vi "Processing Test.vi"(8 "Error In":errorcluster, 11 "File Path Control":path=path "C:/Data/Spectra for Fedor/Ok spectra/300.00000K_175_555_2.10000V_0.00000T_May20-2015__09-37-18_001_052015.tdms") -> (0 "Error Out":errorcluster)   [LabVIEW 2016]
uses:
  LabActor/Post-Processors/Line Detector/Line Detector Configuration.ctl
  <vilib>/Analysis/3filter.llb/Filter Passband Type.ctl
  <vilib>/Analysis/3filter.llb/Bessel Filter (CDB).vi
  Utilities/Fit/Smooth Background CDBL.vi
  <vilib>/addons/Wavelet Analysis/application.llb/WA Denoise (DWT Real Array).vi
  <vilib>/addons/Wavelet Analysis/application.llb/WA Detrend (Array).vi
  <vilib>/addons/Wavelet Analysis/application.llb/WA Multiscale Peak Detection (Array).vi
  <vilib>/Analysis/NI_AALPro.lvlib
  <vilib>/Analysis/NI_AAL_SigProc.lvlib
  <vilib>/Analysis/NI_AALBase.lvlib
  <vilib>/addons/_Advanced Signal Processing/NI_AdvSigProcWA.lvlib
panel:
  out "Waveform Graph":dbl[][](graph)
  in  "ASPT?":bool
  out "# found":i32
  out "error":i32
  in  "Low pass distortion":dbl
  out "XY Graph 6":cluster{dbl[], dbl[]}[](graph)
  in  "User configuration":T1={"Peak width"=30.0, "Background removal"=enum."NONE", "Smoothing"=enum."NONE", "Smooth points"=100.0, "Relative threshold"=0.0, "Peak detector"=enum."Normal", "Bgd points"=100.0} {"Bgd points" format="%#_6p"; "Relative threshold" format="%#_6p"; "Peak width" format="%#_6pHz"}
  in  "Signal channel":string="Signal"
  in  "Frequency channel":string="Frequency"
  in  "group name in":string="p"
  in  "HP F":dbl=0.1 format="%#_6p"
  out "LP  F":dbl=0.001 format="%#_6p"
  in  "Fit?":bool
  in  "Complex":bool
  in  "Deviations":dbl=1.0
  out "variance":dbl format="%.2p"
  out "standard deviation":dbl format="%.2p"
  out "Peak F":dbl format="%#_6pHz"
  out "Points around peak":i32=100
  in  "Peak number":i32
  out "XY Graph 5":cluster{"Array":dbl[], "Array":dbl[]}[](graph)
  out "width":i32=100 min=3
  out "XY Graph 4":cluster{"Y":dbl[], dbl[]}(graph)
  out "XY Graph 3":cluster{"Y":dbl[], "Y":dbl[]}[](graph)
  out "Magnitude":cluster{"Y":dbl[], dbl[]}[](graph)
  out "Phase":cluster{"Y":dbl[], "Unwrapped Phase":dbl[]}[](graph)
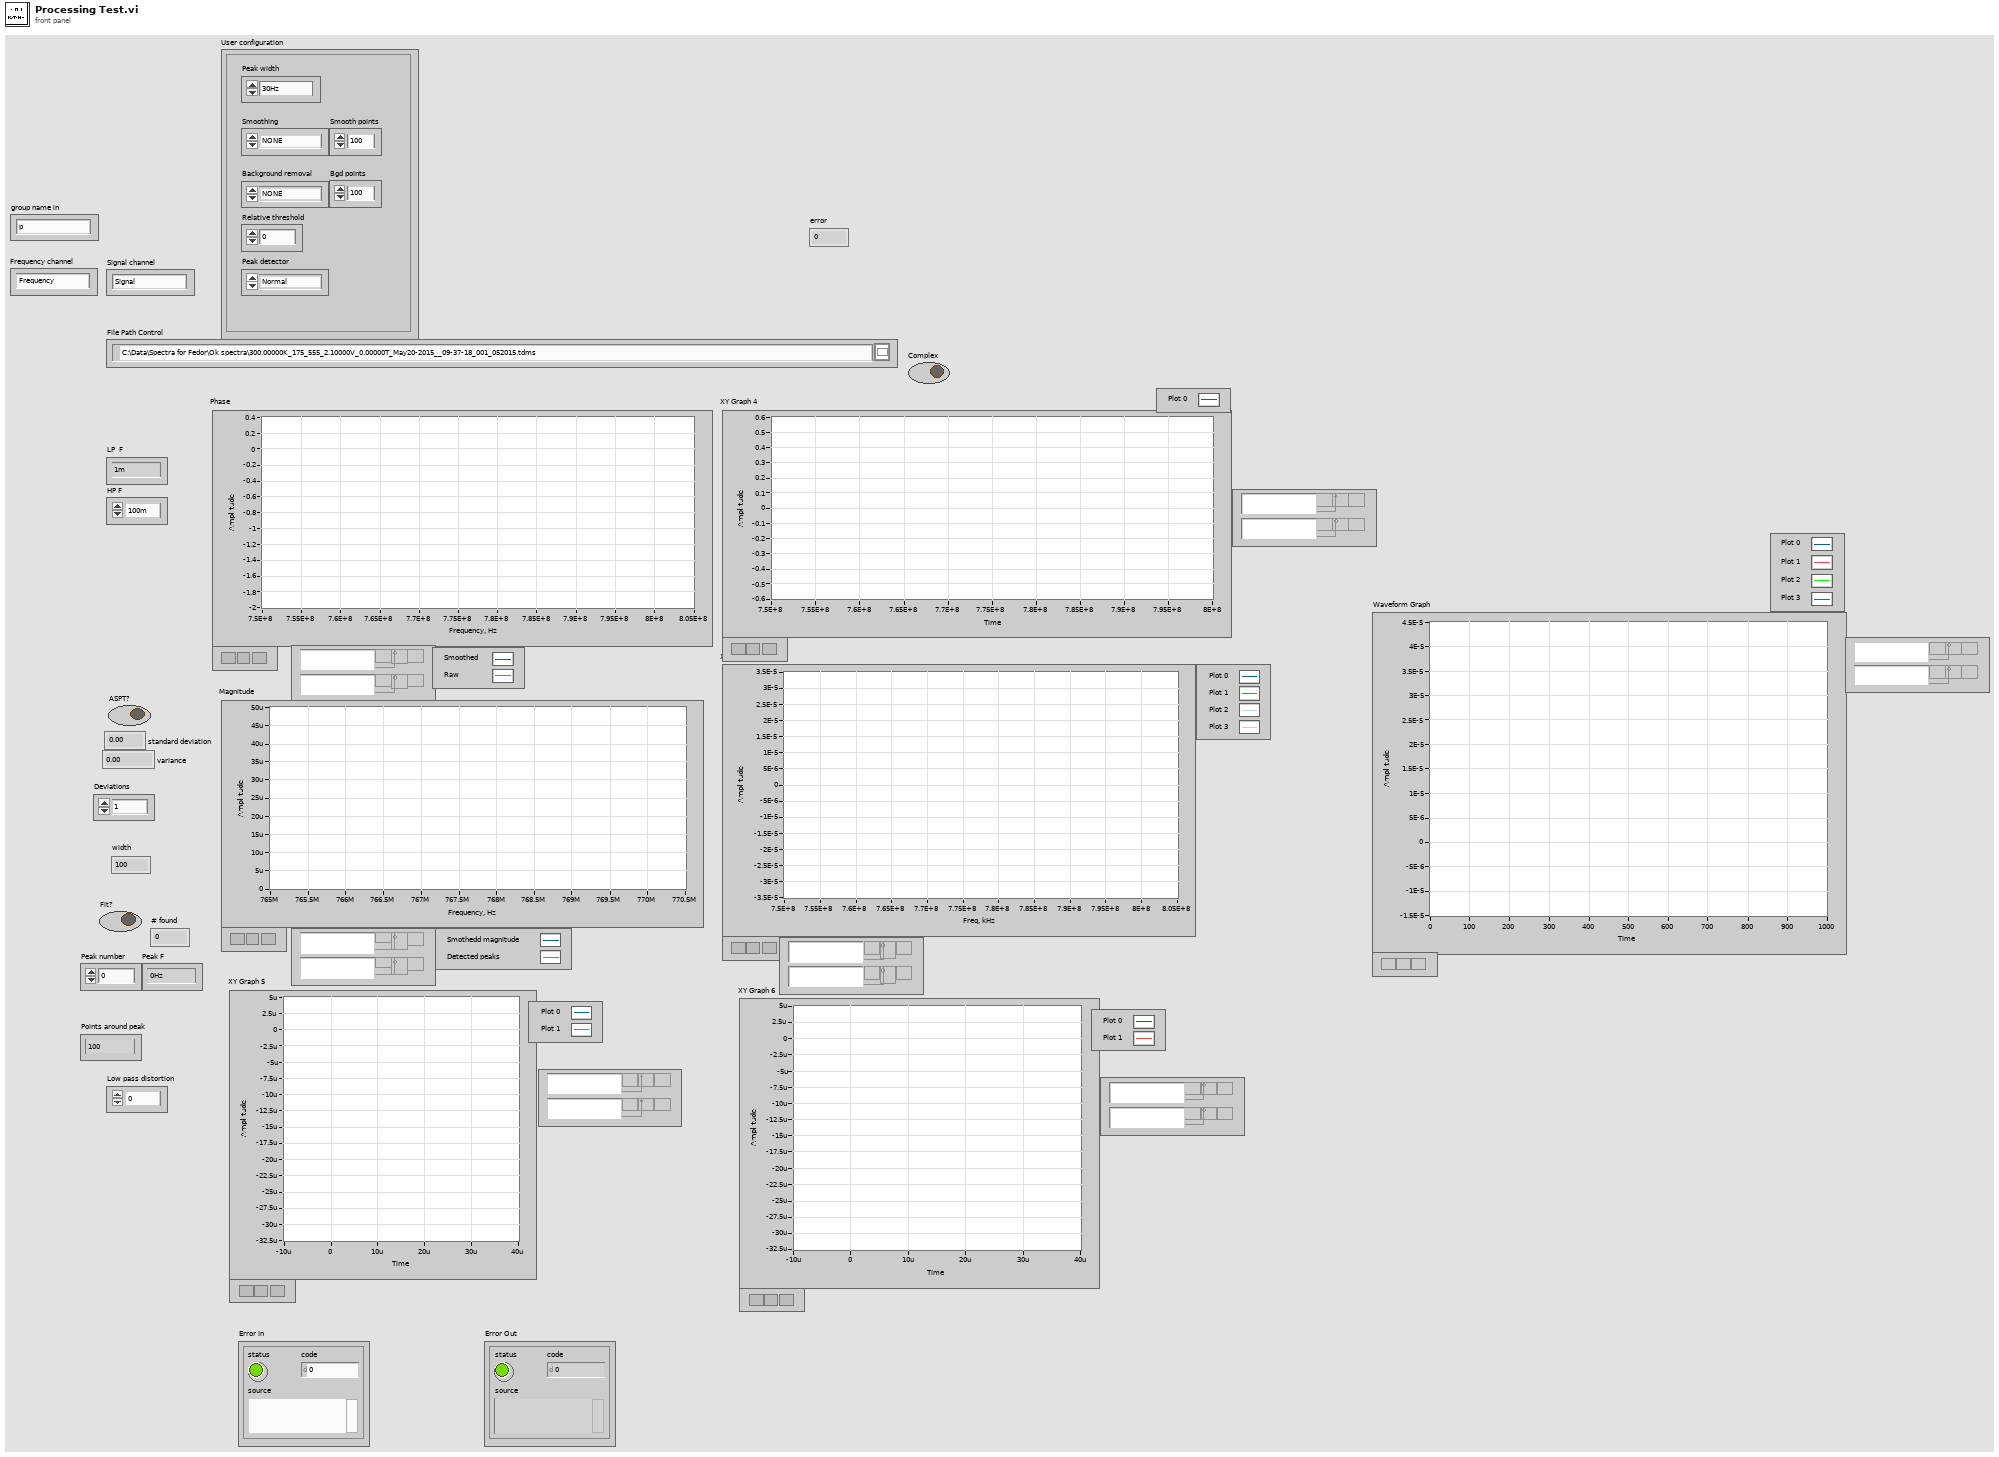
[diagram p1: front panel]
types:
  T1 = typedef "Line Detector Configuration.ctl" = cluster{"Peak width":dbl, "Background removal":enum16{"NONE", "High-pass", "Detrend"}, "Smoothing":enum16{"NONE", "Low-pass", "Denoise"}, "Smooth points":dbl, "Relative threshold":dbl, "Peak detector":enum16{"Normal", "Wavelet", "Wavelet + detrend"}, "Bgd points":dbl}
  T2 = enum16{"open", "open or create", "create or replace", "create", "open (read-only)"}
  T3 = typedef "NI_AALBase.lvlib/Filter Passband Type.ctl" = enum32{"Lowpass", "Highpass", "Bandpass", "Bandstop"}
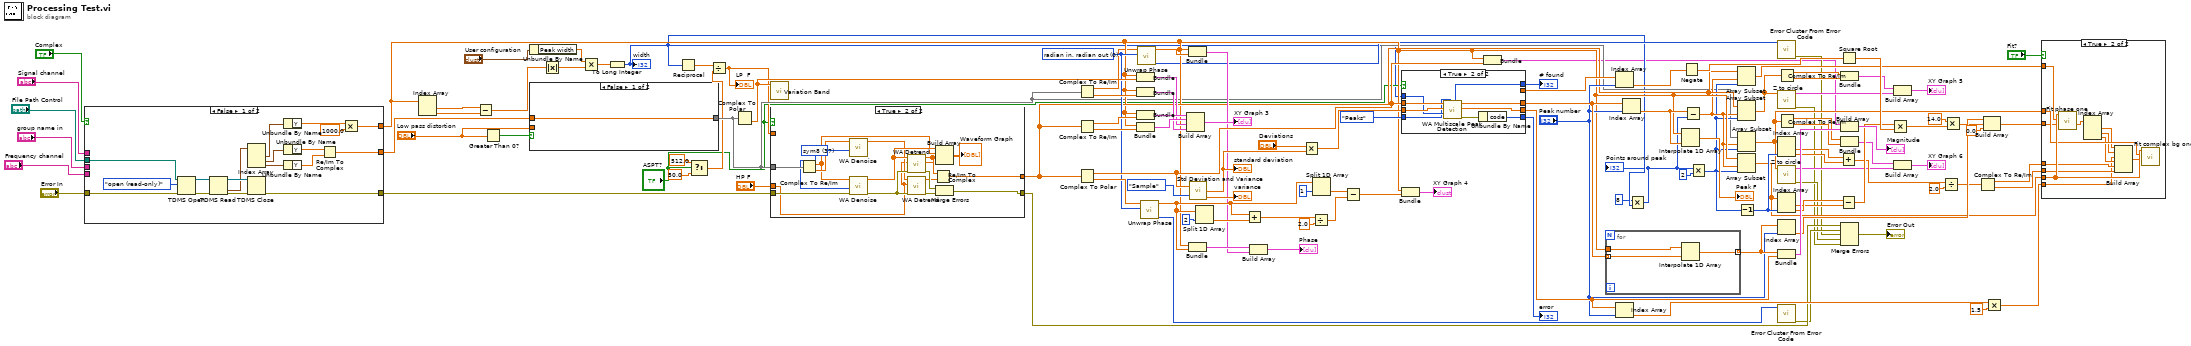
[diagram p0: block diagram]
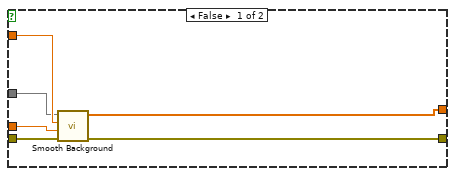
[diagram p2: hidden frame]
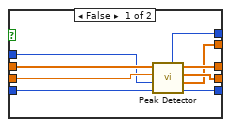
[diagram p3: hidden frame]
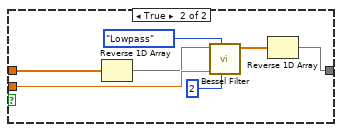
[diagram p4: hidden frame]
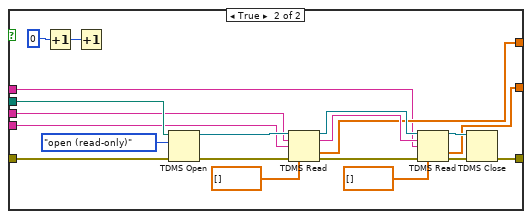
[diagram p6: hidden frame]
diagram:
  w88 = 0 items=["radian in, radian out", "radian in, degree out", "degree in, degree out", "degree in, radian out"] ("phase unit")
  n1 = case shown="False" "Complex" {
    tunnel: "File Path Control" -> [w142 w162]
    tunnel: [w126 w146] -> w48
    tunnel: "group name in" -> [_ w151]
    tunnel: "Frequency channel" -> [_ w150]
    tunnel: [w129 w147] -> w23
    tunnel: "Signal channel" -> [_ w145]
    tunnel: "Error In" -> [w128 w144]
    tunnel: [w127 w143] -> w49
    frame False {
      n2 = TDMS Open(8:w128, 10:T2."open (read-only)" ("operation (0:open)"), 11:w142) -> (0:w139:errorcluster, 3:w140:refnum<k34>)  [unwired: 4 in]
      n3 = TDMS Read(0:w140, 11:w139) -> (4:w138:refnum<k34>, 10:w136:waveform(dbl)[], 15:w137:errorcluster)  [unwired: 6 in, 3 out]
      n4 = Index Array(array=w136) -> (element #1=w135:waveform(dbl), element #2=w133:waveform(dbl), element #3=w134:waveform(dbl))  [unwired: 3 in]
      n5 = TDMS Close(8:w137, 11:w138) -> (0:w127:errorcluster)  [unwired: 1 out]
      n6 = Unbundle By Name(w135) -> ("Y"=w132:dbl[])
      n7 = Unbundle By Name(w133) -> ("Y"=w131:dbl[])
      n8 = Unbundle By Name(w134) -> ("Y"=w130:dbl[])
      n9 = Re/Im To Complex(1:w130, 2:w131) -> (0:w129:cdb[])
      n10 = Multiply(x=w132, y=1000.0) -> (x*y=w126:dbl[])
    }
    frame True {
      n11 = Increment(x=0 ("index")) -> (x+1=w156:i32)
      n12 = Increment(x=w156) -> ()  [unwired: 1 out]
      n13 = TDMS Open(8:w144, 10:T2."open (read-only)" ("operation (0:open)"), 11:w162) -> (0:w159:errorcluster, 3:w160:refnum<k34>)  [unwired: 4 in]
      n14 = TDMS Read(0:w160, 5:w151, 7:w150, 11:w159, 12:dbl[] []) -> (4:w154:refnum<k34>, 6:w152:string, 10:w146:dbl[], 15:w158:errorcluster)  [unwired: 3 in, 2 out]
      n15 = TDMS Read(0:w154, 5:w152, 7:w145, 11:w158, 12:cdb[] []) -> (4:w153:refnum<k34>, 10:w147:cdb[], 15:w155:errorcluster)  [unwired: 3 in, 3 out]
      n16 = TDMS Close(8:w155, 11:w153) -> (0:w143:errorcluster)  [unwired: 1 out]
    }
  }
  n17 = Index Array(array=w48) -> (element #1=w47:dbl, element #2=w46:dbl)  [unwired: 2 in]
  n18 = Subtract(x=w47, y=w46) -> (x-y=w45:dbl)
  n19 = Greater Than 0?(x="Low pass distortion") -> (x > 0?=w25:bool)
  n20 = Unbundle By Name("User configuration") -> ("Peak width"=w43:dbl)
  n21 = case shown="False" w25 {
    tunnel: w23 -> [w163 w170]
    tunnel: [w163 w164] -> w22
    tunnel: "Low pass distortion" -> [_ w167]
    frame False {
    }
    frame True {
      n22 = Reverse 1D Array(array=w170) -> (reversed array=w165:cdb[])
      n23 = call-poly <vilib>:"Bessel Filter.vi"("order"=2, "filter type"=Filter_Passband_Type."Lowpass", "low cutoff freq: fl"=w167, "X"=w165) -> ("Filtered X"=w169:cdb[])  [unwired: 4 in, 1 out]
      n24 = Reverse 1D Array(array=w169) -> (reversed array=w164:cdb[])
    }
  }
  n25 = Absolute Value(x=w45) -> (abs(x)=w42:dbl)
  n26 = Multiply(x=w43, y=w42) -> (x*y=w41:dbl)
  n27 = To Long Integer(number=w41) -> (32bit integer=w4:i32)
  "width" <- w4
  n28 = Reciprocal(x=w4) -> (1/x=w10:dbl)
  n29 = Select(t=512.0, s="ASPT?", f=50.0 ("y")) -> (s? t:f=w7:dbl)
  n30 = Divide(x=w10, y=w7) -> (x/y=w8:dbl)
  "LP  F" <- w8
  n31 = Complex To Polar(r * e^(i*theta)=w22) -> (theta=w11:dbl[])  [unwired: 1 out]
  n32 = call "Variation Band.vi"("Data"=w11) -> ()  [unwired: 11 in]
  n33 = case shown="True" "ASPT?" {
    tunnel: [w176 w191] -> w59
    tunnel: w8 -> [w175 _]
    tunnel: "HP F" -> [w174 w177]
    tunnel: w49 -> [w173 w193]
    tunnel: w22 -> [w172 w183]
    tunnel: [w171 w192] -> w21
    frame False {
      n34 = call-poly "Smooth Background.vi"("Error In"=w173, "HP F"=w174, "LP  F"=w175, "Data"=w172) -> ("Error Out"=w171:errorcluster, "Data out"=w176:cdb[])  [unwired: 6 in]
    }
    frame True {
      w178 = u16 37 items=["db02"=0, "db03"=1, "db04"=2, "db05"=3, "db06"=4, "db07"=5, "db08"=6, "db09"=7, "db10"=8, "db11"=9, "db12"=10, "db13"=11, "db14"=12, "Haar"=13, "bior1_3"=14, "bior1_5"=15, "bior2_2"=16, "bior2_4"=17, "bior2_6"=18, "bior2_8"=19, "bior3_1"=20, "bior3_3"=21, "bior3_5"=22, "bior3_7"=23, "bior3_9"=24, "bior4_4 (FBI)"=25, "bior5_5"=38, "bior6_8"=39, "coif1"=26, "coif2"=27, "coif3"=28, "coif4"=29, "coif5"=30, "sym2"=31, "sym3"=32, "sym4"=33, "sym5"=34, "sym6"=35, "sym7"=36, "sym8"=37] ("wavelet")
      n35 = Complex To Re/Im(x + iy=w183) -> (x=w179:dbl[], y=w181:dbl[])
      n36 = call-poly <vilib>:"WA Denoise.vi"("wavelet"=w178, "signal"=w181) -> ("denoised signal"=w180:dbl[])  [unwired: 8 in, 1 out]
      n37 = call-poly <vilib>:"WA Denoise.vi"("error in (no error)"=w193, "wavelet"=w178, "signal"=w179) -> ("error out"=w184:errorcluster, "denoised signal"=w182:dbl[])  [unwired: 7 in]
      n38 = call-poly <vilib>:"WA Detrend.vi"("error in (no error)"=w184, "threshold frequency"=w177, "signal"=w182) -> ("error out"=w188:errorcluster, "trend signal"=w187:dbl[], "detrended signal"=w189:dbl[])  [unwired: 6 in]
      n39 = call-poly <vilib>:"WA Detrend.vi"("error in (no error)"=w184, "threshold frequency"=w177, "signal"=w180) -> ("error out"=w185:errorcluster, "detrended signal"=w186:dbl[])  [unwired: 6 in, 1 out]
      n40 = Re/Im To Complex(1:w186, 2:w189) -> (0:w191:cdb[])
      n41 = Build Array(w182, w179, w189, w187) -> (→"Waveform Graph":dbl[][])
      n42 = Merge Errors(w188, w185) -> (w192:errorcluster)
    }
  }
  n43 = Complex To Re/Im(x + iy=w22) -> (x=w98:dbl[], y=w99:dbl[])
  n44 = Complex To Re/Im(x + iy=w59) -> (x=w108:dbl[], y=w107:dbl[])
  n45 = Complex To Polar(r * e^(i*theta)=w59) -> (r=w95:dbl[], theta=w114:dbl[])
  n46 = Bundle(w48, w98) -> (w97:cluster{dbl[], dbl[]})  [unwired: 1 in]
  n47 = Bundle(w48, w99) -> (w96:cluster{dbl[], dbl[]})  [unwired: 1 in]
  n48 = Bundle(w48, w108) -> (w122:cluster{dbl[], dbl[]})  [unwired: 1 in]
  n49 = Bundle(w48, w107) -> (w121:cluster{dbl[], dbl[]})  [unwired: 1 in]
  n50 = call <vilib>:"Unwrap Phase.vi"("phase unit"=w88, "Phase"=w11) -> ("error"=w19:i32, "Unwrapped Phase"=w87:dbl[])  [unwired: 8 in]
  n51 = call <vilib>:"Unwrap Phase.vi"("phase unit"=w88, "Phase"=w114) -> ("error"=w20:i32, "Unwrapped Phase"=w109:dbl[])  [unwired: 8 in]
  n52 = Build Array(w122, w121, w97, w96) -> (→"XY Graph 3":cluster{dbl[], dbl[]}[])
  n53 = Bundle(w48, "Unwrapped Phase"=w87) -> (w85:cluster{dbl[], "Unwrapped Phase":dbl[]})  [unwired: 1 in]
  n54 = Bundle(w48, "Unwrapped Phase"=w109) -> (w123:cluster{dbl[], "Unwrapped Phase":dbl[]})  [unwired: 1 in]
  n55 = call <vilib>:"Std Deviation and Variance.vi"("X"=w95, "Weighting (Sample)"=enum16{"Sample", "Population"}."Sample") -> ("standard deviation"=w90:dbl, "variance"=→"variance":dbl)  [unwired: 1 out]
  "standard deviation" <- w90
  n56 = Split 1D Array(array=w109, index=2) -> (second subarray=w117:dbl[])  [unwired: 1 out]
  n57 = Add(x=w109, y=w117) -> (x+y=w116:dbl[])
  n58 = Build Array(w123, w85) -> (→"Phase":cluster{dbl[], "Unwrapped Phase":dbl[]}[])
  n59 = Multiply(x="Deviations", y=w90) -> (x*y=w91:dbl)
  n60 = Divide(x=w116, y=2.0) -> (x/y=w113:dbl[])
  n61 = Split 1D Array(array=w109, index=1) -> (second subarray=w110:dbl[])  [unwired: 1 out]
  n62 = Subtract(x=w110, y=w113) -> (x-y=w112:dbl[])
  n63 = case shown="True" "ASPT?" {
    tunnel: enum32{"Peaks", "Valleys"}."Peaks" ("peaks/valleys") -> [w202 w208]
    tunnel: w95 -> [w201 w211]
    tunnel: w91 -> [w200 w210]
    tunnel: [w199 w205] -> w82
    tunnel: [w198 w206] -> w77
    tunnel: [w197 _] -> w75
    tunnel: w4 -> [w196 w209]
    tunnel: [w195 w203] -> w13
    tunnel: [w194 w207] -> w12
    frame False {
      n64 = call <vilib>:"Peak Detector.vi"("peaks/valleys"=w202, "width"=w196, "threshold"=w200, "X"=w201) -> ("error"=w195:i32, "2nd Derivatives"=w197:dbl[], "Amplitudes"=w199:dbl[], "Locations"=w198:dbl[], "# found"=w194:i32)  [unwired: 3 in]
    }
    frame True {
      n65 = call-poly <vilib>:"WA Multiscale Peak Detection.vi"("peaks/valleys"=w208, "width"=w209, "threshold"=w210, "signal"=w211) -> ("error out"=w204:errorcluster, "amplitude"=w205:dbl[], "location"=w206:dbl[], "number of peaks"=w207:i32)  [unwired: 3 in, 1 out]
      n66 = Unbundle By Name(w204) -> ("code"=w203:i32)
    }
  }
  "error" <- w13
  "# found" <- w12
  n67 = Bundle(w48, w112) -> (→"XY Graph 4":cluster{dbl[], dbl[]})  [unwired: 1 in]
  n68 = Bundle(w48, w95) -> (w1:cluster{dbl[], dbl[]})  [unwired: 1 in]
  n69 = for {
    tunnel: w48 -> [w214]
    tunnel: w77 -> [w213] mode=indexing
    tunnel: [w212] -> w81 mode=indexing
    n70 = Interpolate 1D Array(1:w213, 2:w214) -> (0:w212:dbl)
  }
  n71 = Index Array(array=w75, index="Peak number") -> (element=w74:dbl)
  n72 = Index Array(array=w82, index="Peak number") -> (element=w55:dbl)
  n73 = Index Array(array=w77, index="Peak number") -> (element=w83:dbl)
  n74 = Multiply(x=8, y=w4) -> (x*y=w2:i32)
  "Points around peak" <- w2
  n75 = Interpolate 1D Array(1:w83, 2:w48) -> (0:→"Peak F":dbl)
  n76 = Negate(x=w74) -> (-x=w71:dbl)
  n77 = Subtract(x=w83, y=w2) -> (x-y=w38:dbl)
  n78 = Multiply(x=w2, y=2) -> (x*y=w37:i32)
  n79 = Array Subset(array=w59, index=w38, length=w37) -> (w60:cdb[])
  n80 = Array Subset(array=w59, index=w38, length=w37) -> (w29:cdb[])
  n81 = Array Subset(array=w22, index=w38, length=w37) -> (w31:cdb[])
  n82 = Array Subset(array=w48, index=w38, length=w37) -> (w36:dbl[])
  n83 = Decrement(x=w37) -> (x-1=w80:i32)
  n84 = call <vilib>:"Error Cluster From Error Code.vi"("error code (0)"=w19) -> ("error out"=w16:errorcluster)  [unwired: 8 in]
  n85 = call "Z to circle.vi"("Z"=w29) -> ("Error Out"=w14:errorcluster, "plot"=w27:cluster{"Array":dbl[], "Array":dbl[]})  [unwired: 6 in, 3 out]
  n86 = Index Array(array=w31, index #2=w80) -> (element #1=w70:cdb, element #2=w69:cdb)  [unwired: 1 in]
  n87 = call "Z to circle.vi"("Z"=w31) -> ("Error Out"=w15:errorcluster, "plot"=w30:cluster{"Array":dbl[], "Array":dbl[]})  [unwired: 6 in, 3 out]
  n88 = Index Array(array=w36, index #2=w80) -> (element #1=w78:dbl, element #2=w79:dbl)  [unwired: 1 in]
  n89 = Index Array(array=w81, index="Peak number") -> (element=w67:dbl)
  n90 = Bundle(w81, "amplitude"=w82) -> (w104:cluster{dbl[], "amplitude":dbl[]})  [unwired: 1 in]
  n91 = call <vilib>:"Error Cluster From Error Code.vi"("error code (0)"=w20) -> ("error out"=w17:errorcluster)  [unwired: 8 in]
  n92 = Complex To Re/Im(x + iy=w29) -> (x=w102:dbl[], y=w101:dbl[])
  n93 = Complex To Re/Im(x + iy=w31) -> (x=w34:dbl[], y=w33:dbl[])
  n94 = Add(x=w70, y=w69) -> (x+y=w68:cdb)
  n95 = Subtract(x=w79, y=w78) -> (x-y=w72:dbl)
  n96 = Square Root(x=w71) -> (sqrt(x)=w73:dbl)
  n97 = Bundle(w102, w101) -> (w28:cluster{dbl[], dbl[]})  [unwired: 1 in]
  n98 = Build Array(w1, w104) -> (→"Magnitude":cluster{dbl[], "amplitude":dbl[]}[])
  n99 = Bundle(w34, w33) -> (w35:cluster{dbl[], dbl[]})  [unwired: 1 in]
  n100 = Merge Errors(w21, w17, w16, w15, w14) -> (→"Error Out":errorcluster)
  n101 = Multiply(x=w72, y=w73) -> (x*y=w66:dbl)
  n102 = Build Array(w28, w27) -> (→"XY Graph 5":cluster{"Array":dbl[], "Array":dbl[]}[])
  n103 = Build Array(w35, w30) -> (→"XY Graph 6":cluster{"Array":dbl[], "Array":dbl[]}[])
  n104 = Divide(x=w68, y=2.0) -> (x/y=w63:cdb)
  n105 = Multiply(x=14.0, y=w66) -> (x*y=w40:dbl)
  n106 = Complex To Re/Im(x + iy=w63) -> (x=w62:dbl, y=w61:dbl)
  n107 = Build Array(w67, w40, 0.0 ("element")) -> (w64:dbl[])
  n108 = Multiply(x=w55, y=1.5) -> (x*y=w54:dbl)
  n109 = case shown="True" "Fit?" {
    tunnel: w31 -> [_ w225]
    tunnel: w36 -> [_ w226]
    tunnel: w64 -> [_ w224]
    tunnel: w54 -> [_ w216]
    tunnel: w62 -> [_ w219]
    tunnel: w61 -> [_ w218]
    tunnel: w60 -> [_ w215]
    frame False {
    }
    frame True {
      n110 = call "Fit phase one.vi"("Initial parameters"=w224, "Z"=w215, "X"=w226) -> ("best fit parameters"=w223:dbl[])  [unwired: 7 in, 1 out]
      n111 = Index Array(array=w223) -> (element #1=w222:dbl, element #2=w221:dbl, element #3=w220:dbl)  [unwired: 3 in]
      n112 = Build Array(w222, w221, w216, w220, w219, w218) -> (w217:dbl[])
      n113 = call "Fit complex bg one.vi"("Initial parameters"=w217, "Z"=w225, "X"=w226) -> ()  [unwired: 8 in, 1 out]
    }
  }
